vi "QTrkDLL.vi"() -> ()   [LabVIEW 2011]
panel:
  in  "QTrk DLL Path":path
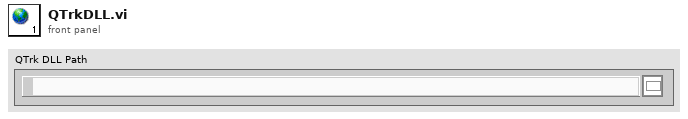
[diagram p1: front panel]
diagram:
